vi "Filter Graphics by File Name.vi"(9 "Keyword":string, 11 "Icon Templates in":T1[](array[typedef])) -> (3 "Icon Templates out":T1[](array[typedef]))   [LabVIEW 2021]
uses:
  <resource>/plugins/NIIconEditor/Controls/Path&Icon.ctl
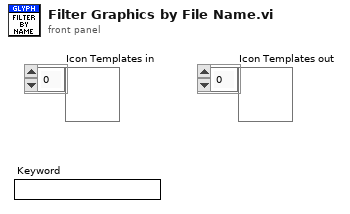
[diagram p1: front panel]
types:
  T1 = typedef "Path&Icon.ctl" = cluster{"Rectangle":cluster{"left":i16, "top":i16, "right":i16, "bottom":i16}, "Path":path, "Image":picture, "Filter":string, "FileName":string}
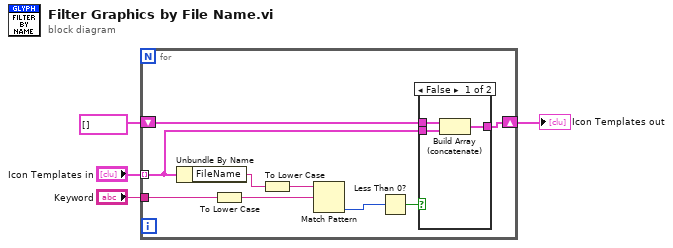
[diagram p0: block diagram]
diagram:
  n1 = for {
    tunnel: "Keyword" -> [w13]
    shift-right: [w9] -> w1
    shift-left: T1[] [] ("ALL available Icons") -> [w10]
    tunnel: "Icon Templates in" -> [w12] mode=indexing
    n2 = Unbundle By Name(w12) -> ("FileName"=w11:string)
    n3 = To Lower Case(string=w13) -> (all lower case string=w5:string)
    n4 = To Lower Case(string=w11) -> (all lower case string=w6:string)
    n5 = Match Pattern(string=w6, regular expression=w5) -> (offset past match=w7:i32)  [unwired: 1 in, 3 out]
    n6 = Less Than 0?(x=w7) -> (x < 0?=w8:bool)
    n7 = case shown="False" w8 {
      tunnel: w12 -> [w16 _]
      tunnel: w10 -> [w15 w17]
      tunnel: [w14 w17] -> w9
      frame False {
        n8 = Build Array (concatenate)(w15, w16) -> (w14:T1[])
      }
      frame True {
      }
    }
  }
  "Icon Templates out" <- w1
